vi "fgv_do_speed.vi"(7 "cmd":enum16{"speed", "steer", "close", "ini"}(ring), 10 "steer":u16, 11 "speed":u16) -> ()   [LabVIEW 2017]
uses:
  <vilib>/myRIO/Common/Instrument Driver Framework/Utilities/typedefs/Analog Scaling Constants.ctl
  <vilib>/myRIO/Common/Instrument Driver Framework/Utilities/typedefs/Analog Scaling Constants List.ctl
  <vilib>/myRIO/Common/Instrument Driver Framework/myRIO v1.0/AO/typedefs/AO Channels Enum.ctl
  <vilib>/myRIO/Common/Instrument Driver Framework/myRIO v1.0/AO/typedefs/AO Channels List.ctl
  <vilib>/myRIO/Common/Instrument Driver Framework/Utilities/typedefs/Generic FPGA Reference.ctl
  <vilib>/myRIO/Common/Instrument Driver Framework/Utilities/typedefs/myRIO v1.0 Reference.ctl
  <vilib>/myRIO/Common/Instrument Driver Framework/Utilities/typedefs/Hardware Version Enum.ctl
  <vilib>/myRIO/Common/Instrument Driver Framework/Utilities/typedefs/myRIO Generic Hardware Reference.ctl
  <vilib>/myRIO/Instrument Drivers/Onboard IO/AO/typedefs/AO Reference.ctl
  <vilib>/myRIO/Instrument Drivers/Onboard IO/AO/AO.lvlib
  <vilib>/myRIO/Instrument Drivers/Onboard IO/AO/vis/myRIO AO Open.xnode
  <vilib>/myRIO/Common/Instrument Driver Framework/myRIO v1.0/AO/vis/myRIO v1.1 Open AO.vi
  <vilib>/userdefined/High Color/nirio_resource_hc.ctl
  <vilib>/myRIO/Instrument Drivers/Onboard IO/PWM/typedefs/PWM Configuration.ctl
  <vilib>/myRIO/Instrument Drivers/Onboard IO/PWM/PWM.lvlib
  <vilib>/myRIO/Common/Instrument Driver Framework/myRIO v1.0/PWM/typedefs/PWM Channels Enum.ctl
  <vilib>/myRIO/Instrument Drivers/Onboard IO/PWM/typedefs/PWM Reference.ctl
  <vilib>/myRIO/Instrument Drivers/Onboard IO/PWM/vis/myRIO PWM Open.xnode
  <vilib>/myRIO/Common/Instrument Driver Framework/myRIO v1.0/PWM/vis/myRIO v1.1 Open PWM.vi
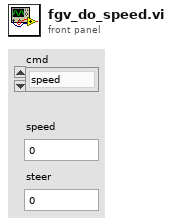
[diagram p1: front panel]
types:
  T1 = typedef "nirio_resource_hc.ctl" = tag
  T2 = typedef "Hardware Version Enum.ctl" = enum16{"Unknown", "myRIO-1900", "myRIO-1950", "roboRIO", "NI ELVIS RIO CM"}
  T3 = typedef "PWM.lvlib/PWM Reference.ctl" = cluster{"myRIO Reference":T4, "PWM Channels Enum":T7, "PWM Configuration":T8}
  T4 = typedef "myRIO Generic Hardware Reference.ctl" = cluster{"myRIO Model":T2, "myRIO Hardware Reference":T5}
  T5 = typedef "myRIO v1.0 Reference.ctl" = cluster{"Generic FPGA Reference":T6, "Allow multiple opens":bool}
  T6 = typedef "Generic FPGA Reference.ctl" = refnum<k20>
  T7 = typedef "PWM Channels Enum.ctl" = enum16{"Not Connected", "C/PWM0", "C/PWM1", "A/PWM0", "A/PWM1", "A/PWM2", "B/PWM0", "B/PWM1", "B/PWM2", "PWM/PWM0", "PWM/PWM1", "PWM/PWM2", "PWM/PWM3", "PWM/PWM4", "PWM/PWM5", "PWM/PWM6", "PWM/PWM7", "PWM/PWM8", "PWM/PWM9"}
  T8 = typedef "PWM.lvlib/PWM Configuration.ctl" = cluster{"Frequency":dbl, "Duty Cycle":dbl}
  T9 = typedef "AO.lvlib/AO Reference.ctl" = cluster{"myRIO Reference":T4, "AO Channel List":T10, "AO Scaling Constant List":T12}
  T10 = typedef "AO Channels List.ctl" = T11[]
  T11 = typedef "AO Channels Enum.ctl" = enum16{"Not Connected", "AudioOut/Left", "AudioOut/Right", "C/AO0", "C/AO1", "A/AO0", "A/AO1", "B/AO0", "B/AO1"}
  T12 = typedef "Analog Scaling Constants List.ctl" = T13[]
  T13 = typedef "Analog Scaling Constants.ctl" = cluster{"LSB Weight (Volts)":dbl, "Offset (Volts)":dbl, "Signed?":bool}
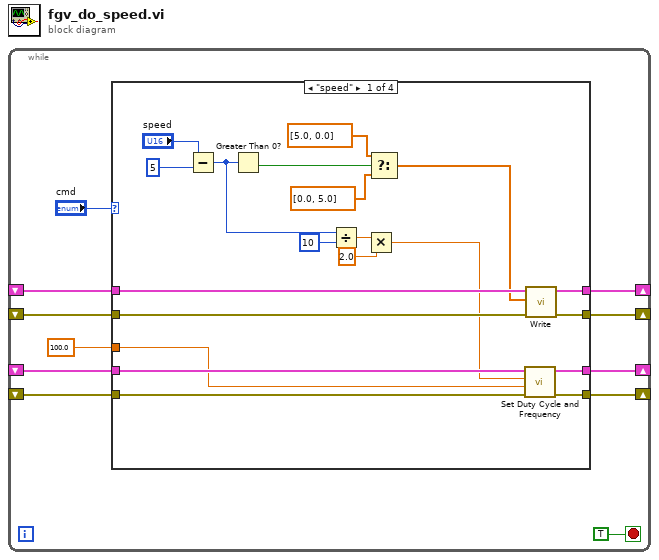
[diagram p0: block diagram]
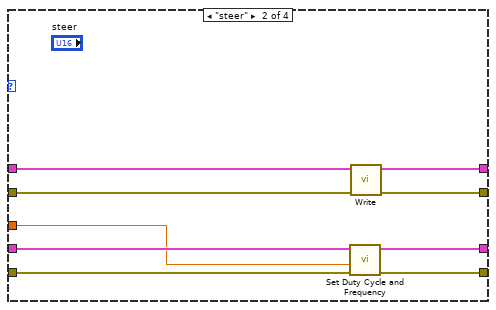
[diagram p2: hidden frame]
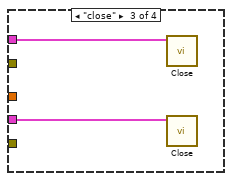
[diagram p3: hidden frame]
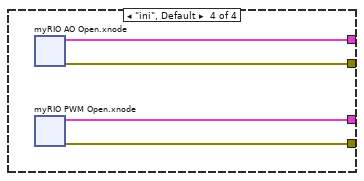
[diagram p4: hidden frame]
diagram:
  n1 = while {
    shift-right: [w9] -> _
    shift-left: _ -> [w7]
    shift-right: [w8] -> _
    shift-left: _ -> [w6]
    shift-right: [w5] -> _
    shift-left: _ -> [w3]
    shift-right: [w4] -> _
    shift-left: _ -> [w2]
    stop <- TRUE stop-if-true
    n2 = case shown="\"speed\"" "cmd" {
      tunnel: [w31 w40 _ w46] -> w9
      tunnel: [w30 w39 _ w45] -> w8
      tunnel: w7 -> [w29 w38 w41 _]
      tunnel: w6 -> [w28 w37 _ _]
      tunnel: [w26 w35 _ w44] -> w5
      tunnel: [w27 w36 _ w43] -> w4
      tunnel: w3 -> [w25 w34 w42 _]
      tunnel: w2 -> [w24 w33 _ _]
      tunnel: 100.0 ("Frequency [Hz]") -> [w23 w32 _ _]
      frame "speed" {
        n3 = Subtract(x="speed", y=u16 5) -> (x-y=w20:u16)
        n4 = Greater Than 0?(x=w20) -> (x > 0?=w15:bool)
        n5 = Divide(x=w20, y=u16 10) -> (x/y=w17:dbl)
        n6 = Multiply(x=w17, y=2.0) -> (x*y=w19:dbl)
        n7 = Select(t=dbl[] [5.0, 0.0], s=w15, f=dbl[] [0.0, 5.0]) -> (s? t:f=w12:dbl[])
        n8 = call <vilib>:"Set Duty Cycle and Frequency.vi"("error in (no error)"=w24, "Frequency [Hz]"=w23, "Duty Cycle"=w19, "PWM Ref In"=w25) -> ("error out"=w27:errorcluster, "PWM Ref Out"=w26:T3)  [unwired: 5 in]
        n9 = call <vilib>:"Write.vi"("error in (no error)"=w28, "Values"=w12, "AO Ref In"=w29) -> ("error out"=w30:errorcluster, "AO Ref Out"=w31:T9)  [unwired: 6 in]
      }
      frame "steer" {
        n10 = call <vilib>:"Set Duty Cycle and Frequency.vi"("error in (no error)"=w33, "Frequency [Hz]"=w32, "PWM Ref In"=w34) -> ("error out"=w36:errorcluster, "PWM Ref Out"=w35:T3)  [unwired: 6 in]
        n11 = call <vilib>:"Write.vi"("error in (no error)"=w37, "AO Ref In"=w38) -> ("error out"=w39:errorcluster, "AO Ref Out"=w40:T9)  [unwired: 7 in]
      }
      frame "close" {
        n12 = call <vilib>:"Close.vi"("AO Ref In"=w41) -> ()  [unwired: 10 in, 1 out]
        n13 = call <vilib>:"Close.vi"("PWM Ref In"=w42) -> ()  [unwired: 10 in, 1 out]
      }
      frame "ini", Default {
        n14 = xnode "myRIO AO Open.xnode"() -> ("error out"=w45:errorcluster, "AO Ref Out"=w46:T9)  [unwired: 3 in]
        n15 = xnode "myRIO PWM Open.xnode"() -> ("error out"=w43:errorcluster, "PWM Ref Out"=w44:T3)  [unwired: 3 in]
      }
    }
  }
